vi "AnalysisSettingsToFile.vi"(8 "ErrorIn":errorcluster, 9 "Save to file?":bool, 11 "AnalysisSettingsString":string) -> (0 "ErrorOut":errorcluster)   [LabVIEW 2019]
uses:
  VibrationDiagnosisDesktopApp/mainVIs/DialogsVIs/AnalysisSettings.ctl
  analyzeAccelerationDataVIs/calculateFaultIndicatorsVIs/Thresholds.ctl
  analyzeAccelerationDataVIs/calculateFaultIndicatorsVIs/FaultParameter.ctl
  aquireAccelerationDataVIs/Accelerometer.ctl
  utilities/FGVAction.ctl
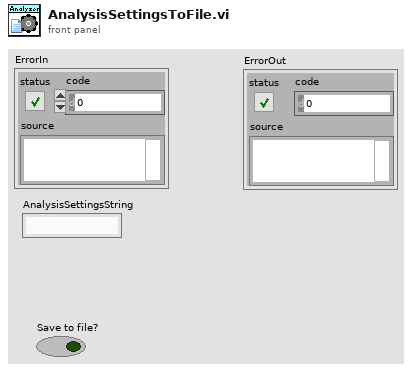
[diagram p1: front panel]
types:
  T1 = typedef "AnalysisSettings.ctl" = cluster{"Fault Thresholds":T2, "Analysis series name":string, "Save data analysis?":bool, "F-Band Size":i32, "OrderAnalysis?":bool, "Accelerometer":T4, "fs [Hz]":dbl, "Pulse per revolution":u16, "FFT-Parameters":cluster{"averaging mode":enum16{"No averaging", "Vector averaging", "RMS averaging", "Peak hold"}, "weighting mode":enum16{"Linear", "Exponential"}, "number of averages":u32}, "O-WindowPowerSpectrum":u32, "O-SpectrumAveraging":enum16{"No averaging", "Vector averaging", "RMS averaging", "Peak hold"}, "O-MaxOrder":dbl, "O-Resolution":dbl, "O-BandSize":dbl, "FrameLength [s]":dbl, "Aq.FrameLength [ms]":i64, "FilterOrder":i32, "Sensitivity [V/g]":dbl[]}
  T2 = typedef "Thresholds.ctl" = cluster{"Parameters labels":T3[], "Parameters thresholds":dbl[], "Freqs and thresholds":dbl[][], "Orders and thresholds":dbl[][]}
  T3 = typedef "FaultParameter.ctl" = enum16{"Kurtosis", "RMS", "Crest factor"}
  T4 = typedef "Accelerometer.ctl" = enum16{"None", "MPU6050", "MMA7351"}
  T5 = enum16{"open", "replace", "create", "open or create", "replace or create", "replace or create with confirmation"}
  T6 = typedef "FGVAction.ctl" = enum16{"Read", "Write"}
  T7 = typedef "AnalyzerSettings.ctl" = cluster{"Create NS Timeout Code":i32, "Destroy NS Timeout Code":i32, "All threads":T8[], "Connected to app?":bool, "AnalysisSettings":T1}
  T8 = typedef "AThreads.ctl" = enum16{"UI", "analyzeAccelerationData", "aquireAccelerationData", "communicateWebServices", "TDMSmanager", "aquireTachoSignal"}
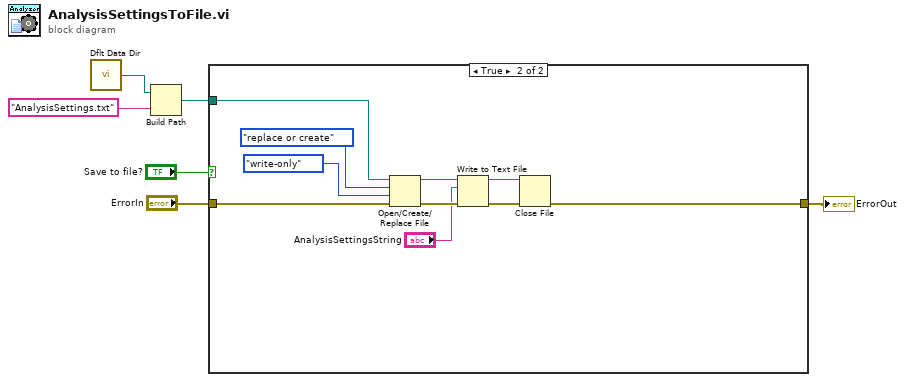
[diagram p0: block diagram]
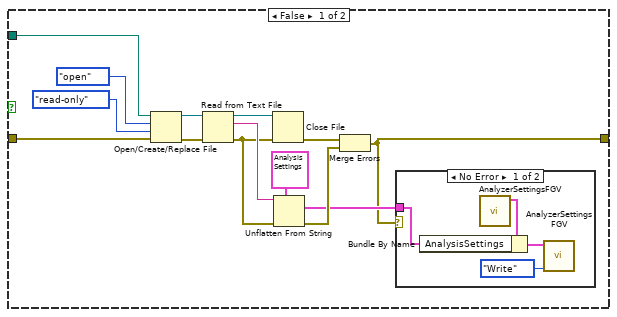
[diagram p2: hidden frame]
diagram:
  n1 = call <vilib>:"Dflt Data Dir.vi"() -> ("App:Default Data Directory"=w4:path)
  n2 = Build Path(base path=w4, name or relative path="AnalysisSettings.txt") -> (appended path=w3:path)
  n3 = case shown="True" "Save to file?" {
    tunnel: "ErrorIn" -> [w18 w34]
    tunnel: w3 -> [w15 w33]
    tunnel: [w7 w25] -> w2
    frame False {
      n4 = Open/Create/Replace File(file path (use dialog)=w15, error in=w18, operation (0:open)=T5."open", access (0:read/write)=enum16{"read/write", "read-only", "write-only"}."read-only") -> (refnum out=w20:refnum<file>, error out=w17:errorcluster)  [unwired: 2 in, 1 out]
      n5 = Read from Text File(file (use dialog)=w20, error in=w17) -> (refnum out=w19:refnum<file>, text=w12:string, error out=w10:errorcluster)  [unwired: 2 in, 1 out]
      n6 = Close File(refnum=w19, error in=w10) -> (error out=w16:errorcluster)  [unwired: 1 out]
      n7 = Unflatten From String(type=T1 {"Fault Thresholds"={"Parameters labels"=[], "Parameters thresholds"=[], "Freqs and thresholds"=[], "Orders and thresholds"=[]}, "Analysis series name"="Analiza", "Save data analysis?"=TRUE, "F-Band Size"=20, "OrderAnalysis?"=FALSE, "Accelerometer"=enum."MPU6050", "fs [Hz]"=2000.0, "Pulse per revolution"=0, "FFT-Parameters"={"averaging mode"=enum."No averaging", "weighting mode"=enum."Linear", "number of averages"=0}, "O-WindowPowerSpectrum"=0, "O-SpectrumAveraging"=enum."No averaging", "O-MaxOrder"=0.0, "O-Resolution"=0.0, "O-BandSize"=0.0, "FrameLength [s]"=1.0, "Aq.FrameLength [ms]"=0, "FilterOrder"=0, "Sensitivity [V/g]"=[]} ("AnalysisSettings"), binary string=w12, error in (no error)=w10) -> (value=w8:T1, error out=w9:errorcluster)  [unwired: 2 in, 1 out]
      n8 = Merge Errors(w16, w9) -> (w7:errorcluster)
      n9 = case shown="No Error" w7 {
        tunnel: w8 -> [w23 _]
        frame No Error {
          n10 = call "AnalyzerSettingsFGV.vi"() -> ("AnalyzerSettingsOut"=w24:T7)  [unwired: 11 in]
          n11 = Bundle By Name(cluster=w24, "AnalysisSettings"=w23) -> (w22:T7)
          n12 = call "AnalyzerSettingsFGV.vi"("FGVAction (Read)"=FGVAction."Write", "AnalyzerSettingsIn"=w22) -> ()  [unwired: 9 in, 1 out]
        }
        frame Error {
        }
      }
    }
    frame True {
      n13 = Open/Create/Replace File(file path (use dialog)=w33, error in=w34, operation (0:open)=T5."replace or create", access (0:read/write)=enum16{"read/write", "read-only", "write-only"}."write-only") -> (refnum out=w30:refnum<file>, error out=w29:errorcluster)  [unwired: 2 in, 1 out]
      n14 = Write to Text File(file (use dialog)=w30, text="AnalysisSettingsString", error in=w29) -> (refnum out=w27:refnum<file>, error out=w26:errorcluster)  [unwired: 1 in, 1 out]
      n15 = Close File(refnum=w27, error in=w26) -> (error out=w25:errorcluster)  [unwired: 1 out]
    }
  }
  "ErrorOut" <- w2
